vi "Gravity Loading (Point).vi"(8 "error in (no error)":errorcluster, 9 "gravity":dbl[](array[numeric]), 10 "joint positions":dbl[](array[numeric]), 11 "serial arm in":refnum<class "NI_Robotics_Serial Robot Arm.lvclass">) -> (0 "error out":errorcluster, 2 "torques":dbl[](array[numeric]), 3 "serial arm out":refnum<class "NI_Robotics_Serial Robot Arm.lvclass">)   [LabVIEW 2017, in "NI_Kinematics.lvlib"]
doc: "Calculates the torque that gravity applies to each joint of a robotic arm. Wire data to the <B>joint positions</B> input to determine the polymorphic instance to use or manually select the instance. \n\n<B>.m file:</B> gravload"
uses:
  <vilib>/robotics/Kinematics/NI_Kinematics.lvlib
  <vilib>/robotics/Kinematics/Robot/NI_Robotics_Serial Robot Arm.lvclass
  <vilib>/robotics/Kinematics/dyn/Inverse Dynamics (Point).vi
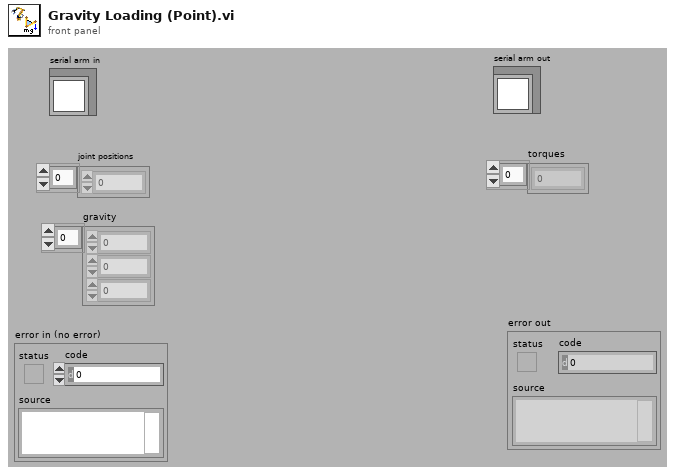
[diagram p1: front panel]
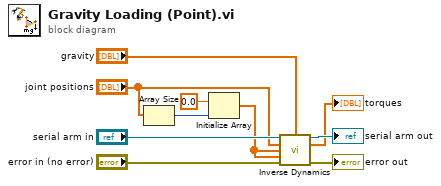
[diagram p0: block diagram]
diagram:
  n1 = Array Size(array="joint positions") -> (size(s)=w6:i32)
  n2 = Initialize Array(0.0 ("element"), w6) -> (w5:dbl[])
  n3 = call-poly <vilib>:"Inverse Dynamics.vi"("serial arm in"="serial arm in", "gravity"="gravity", "joint positions"="joint positions", "joint velocities"=w5, "joint accelerations"=w5, "error in (no error)"="error in (no error)") -> ("serial arm out"=→"serial arm out":refnum<class "NI_Robotics_Serial Robot Arm.lvclass">, "required torques"=→"torques":dbl[], "error out"=→"error out":errorcluster)  [unwired: 7 in]
